vi "LookAheadPoint.vi"(8 "Robot":cluster{"x":dbl, "y":dbl}, 9 "Spacing":dbl, 10 "LookAhead":dbl, 11 "Path":cluster{"x":dbl, "y":dbl}[](array[cluster])) -> (2 "Index":i32, 3 "Point":cluster{"x":dbl, "y":dbl})   [LabVIEW 2016]
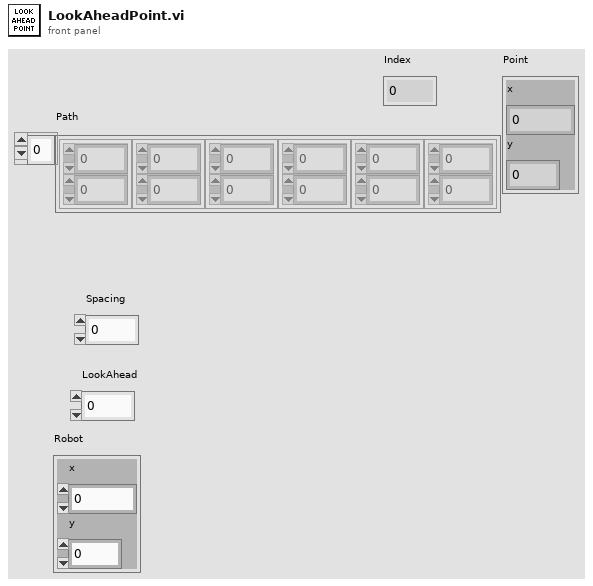
[diagram p1: front panel]
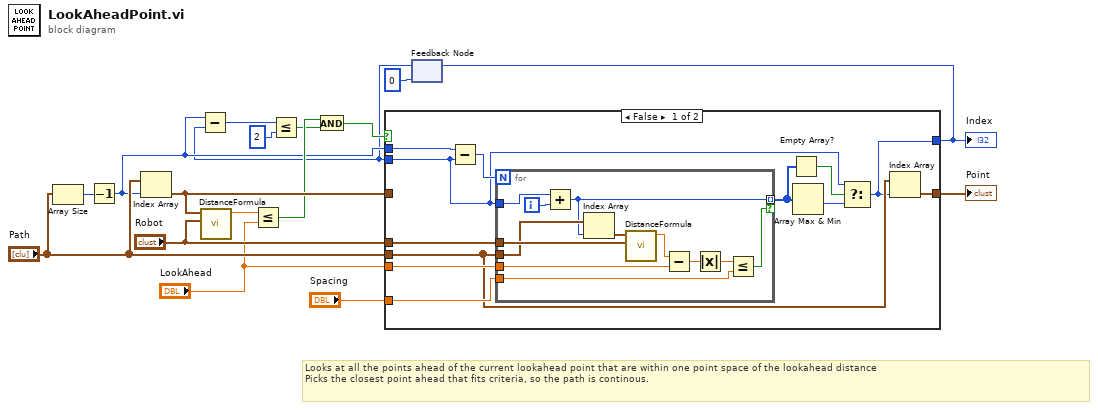
[diagram p0: block diagram]
diagram:
  # "Looks at all the points ahead of the current lookahead point that are within one point space of the lookahead distance\nPicks the closest point ahead that fits criteria, so the path is continous."
  n1 = Array Size(array="Path") -> (size(s)=w16:i32)
  n2 = Decrement(x=w16) -> (x-1=w5:i32)
  n3 = Index Array(array="Path", index=w5) -> (element=w11:cluster{"x":dbl, "y":dbl})
  n4 = call "DistanceFormula.vi"("Point 2"="Robot", "Point 1"=w11) -> ("Distance"=w9:dbl)  [unwired: 9 in]
  n5 = Less Or Equal?(x=w9, y="LookAhead") -> (x <= y?=w7:bool)
  n6 = feedback #1(0) -> (w4:i32)
  n7 = Subtract(x=w5, y=w4) -> (x-y=w3:i32)
  n8 = Less Or Equal?(x=w3, y=2) -> (x <= y?=w1:bool)
  n9 = And(x=w7, y=w1) -> (x .and. y?=w6:bool)
  n10 = case shown="False" w6 {
    tunnel: "LookAhead" -> [w29 _]
    tunnel: [w28 w43] -> w17
    tunnel: "Path" -> [w23 _]
    tunnel: "Robot" -> [w27 _]
    tunnel: [w18 w42] -> w13
    tunnel: w11 -> [_ w43]
    tunnel: w5 -> [w26 w42]
    tunnel: "Spacing" -> [w24 _]
    tunnel: w4 -> [w19 _]
    frame False {
      n11 = Subtract(x=w26, y=w19) -> (x-y=w25:i32)
      n12 = for {
        N: w25 -> [_]
        tunnel: w23 -> [w37]
        tunnel: w27 -> [w41]
        tunnel: w29 -> [w39]
        tunnel: w19 -> [w35]
        tunnel: w24 -> [w32]
        tunnel: [w31] -> w22 mode=indexing if=w30
        i -> [w36]
        n13 = Add(x=w35, y=w36) -> (x+y=w31:i32)
        n14 = Index Array(array=w37, index=w31) -> (element=w34:cluster{"x":dbl, "y":dbl})
        n15 = call "DistanceFormula.vi"("Point 2"=w41, "Point 1"=w34) -> ("Distance"=w40:dbl)  [unwired: 9 in]
        n16 = Subtract(x=w40, y=w39) -> (x-y=w38:dbl)
        n17 = Absolute Value(x=w38) -> (abs(x)=w33:dbl)
        n18 = Less Or Equal?(x=w33, y=w32) -> (x <= y?=w30:bool)
      }
      n19 = Empty Array?(array=w22) -> (empty?=w21:bool)
      n20 = Array Max & Min(array=w22) -> (min value=w20:i32)  [unwired: 3 out]
      n21 = Select(t=w19, s=w21, f=w20) -> (s? t:f=w18:i32)
      n22 = Index Array(array=w23, index=w18) -> (element=w28:cluster{"x":dbl, "y":dbl})
    }
    frame True {
    }
  }
  "Point" <- w17
  "Index" <- w13
  n23 = feedback-in #1(w13) -> ()
